vi "Get ChromaDB Folder.vi"(11 "ChromaDB Folder in":path caption="Embedding Model URL in") -> (3 "ChromaDB Folder out":path)   [LabVIEW 2023, in "LabVIEW RAG.lvlib"]
uses:
  LabVIEW RAG.lvlib
  AI RAG Globals.vi
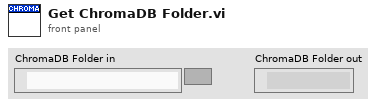
[diagram p1: front panel]
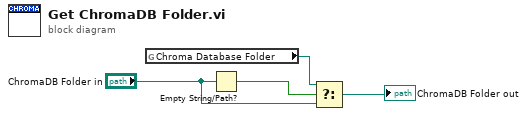
[diagram p0: block diagram]
diagram:
  n1 = global read "AI RAG Globals.vi" "Chroma Database Folder"() -> (w4:path)
  n2 = Empty String/Path?(string/path="ChromaDB Folder in") -> (empty?=w3:bool)
  n3 = Select(t=w4, s=w3, f="ChromaDB Folder in") -> (s? t:f=→"ChromaDB Folder out":path)
